vi "Execution Command.vi"(8 "error in (no error)":errorcluster, 11 "Block Command":T1) -> (0 "error out":errorcluster)   [LabVIEW 2022 SP3, in "FlexBlocks Support.lvlib"]
uses:
  FlexBlocks Support.lvlib
  <vilib>/event_ctls.llb/usereventprio.ctl
  Block Command.ctl
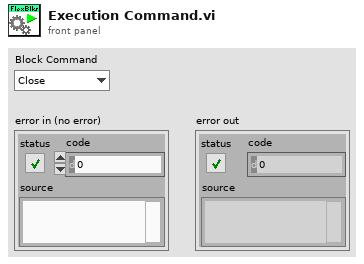
[diagram p1: front panel]
types:
  T1 = typedef "FlexBlocks Support.lvlib/Block Command.ctl" = enum16{"Close", "Init", "Step", "Run", "Pause"}
  T2 = typedef "FlexBlocks Support.lvlib/Execution Events.ctl" = cluster{"Registration":refnum<user-event>, "Init":refnum<user-event>, "Run":refnum<user-event>, "Step":refnum<user-event>, "Stop":refnum<user-event>, "Close":refnum<user-event>, "Block Status":refnum<user-event>}
  T3 = typedef "usereventprio.ctl" = enum32{"high priority", "normal priority"}
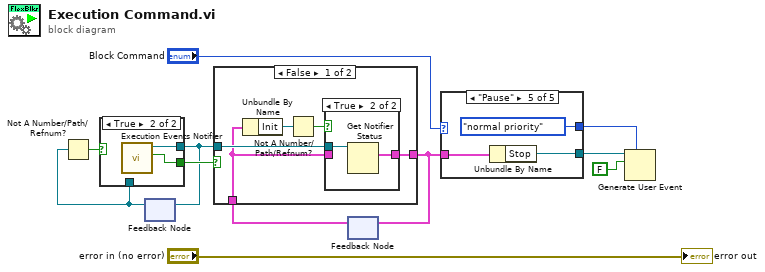
[diagram p0: block diagram]
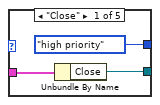
[diagram p2: hidden frame]
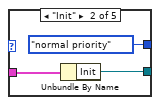
[diagram p3: hidden frame]
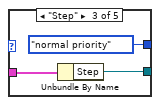
[diagram p4: hidden frame]
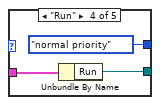
[diagram p5: hidden frame]
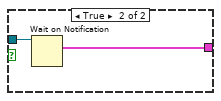
[diagram p7: hidden frame]
diagram:
  n1 = feedback #1() -> (w10:refnum<notifier>)  [unwired: 1 in]
  n2 = Not A Number/Path/Refnum?(number/path/refnum=w10) -> (NaN/Path/Refnum?=w11:bool)
  n3 = case shown="True" w11 {
    tunnel: [w12 w14] -> w8
    tunnel: w10 -> [w12 _]
    tunnel: [_ w13] -> w9
    frame False {
    }
    frame True {
      n4 = call "Execution Events Notifier.vi"() -> ("created new?"=w13:bool, "Events Notifier"=w14:refnum<notifier>)  [unwired: 10 in]
    }
  }
  n5 = feedback-in #1(w8) -> ()
  n6 = feedback #2() -> (w7:T2)  [unwired: 1 in]
  n7 = case shown="False" w9 {
    tunnel: w8 -> [w17 w24]
    tunnel: [w16 w23] -> w6
    tunnel: w7 -> [w15 _]
    frame False {
      n8 = Unbundle By Name(w15) -> ("Init"=w19:refnum<user-event>)
      n9 = Not A Number/Path/Refnum?(number/path/refnum=w19) -> (NaN/Path/Refnum?=w18:bool)
      n10 = case shown="True" w18 {
        tunnel: w17 -> [_ w22]
        tunnel: [w20 w21] -> w16
        tunnel: w15 -> [w20 _]
        frame False {
        }
        frame True {
          n11 = Get Notifier Status(notifier=w22) -> (current notification=w21:T2)  [unwired: 1 in, 4 out]
        }
      }
    }
    frame True {
      n12 = Wait on Notification(notifier=w24) -> (notification=w23:T2)  [unwired: 3 in, 3 out]
    }
  }
  n13 = feedback-in #2(w6) -> ()
  n14 = case shown="\"Pause\"" "Block Command" {
    tunnel: w6 -> [w27 w30 w33 w36 w39]
    tunnel: [w26 w29 w32 w35 w38] -> w4
    tunnel: [usereventprio."high priority" ("priority (normal)") usereventprio."normal priority" ("priority (normal)") usereventprio."normal priority" ("priority (normal)") usereventprio."normal priority" ("priority (normal)") usereventprio."normal priority" ("priority (normal)")] -> w2
    frame "Close" {
      n15 = Unbundle By Name(w27) -> ("Close"=w26:refnum<user-event>)
    }
    frame "Init" {
      n16 = Unbundle By Name(w30) -> ("Init"=w29:refnum<user-event>)
    }
    frame "Step" {
      n17 = Unbundle By Name(w33) -> ("Step"=w32:refnum<user-event>)
    }
    frame "Run" {
      n18 = Unbundle By Name(w36) -> ("Run"=w35:refnum<user-event>)
    }
    frame "Pause" {
      n19 = Unbundle By Name(w39) -> ("Stop"=w38:refnum<user-event>)
    }
  }
  n20 = Generate User Event(priority (normal)=w2, user event=w4, event data cluster=FALSE ("event data")) -> ()  [unwired: 1 in, 2 out]
  "error out" <- "error in (no error)"
